vi "Clean-up List of Observables.vi"(1 "Obsv to check":string[](array[string]) caption="Quality of Run Check") -> (0 "Array":T1(array[cluster]))   [LabVIEW 2020, in "TALOS.lvlib" / "Scheduler.lvlib"]
uses:
  Scheduler.lvlib
  6c034efd-64e3-466f-95ca-04aa63bb7247.vi
  <vilib>/Comparison/Equal/Equal Functor/Equal Functor.lvclass
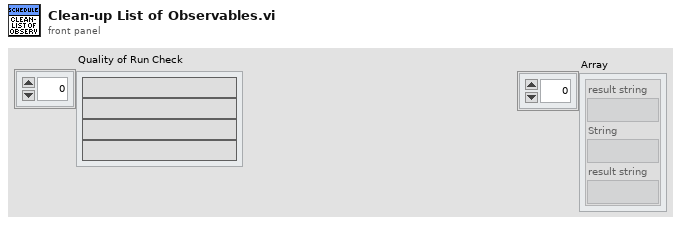
[diagram p1: front panel]
types:
  T1 = cluster{"result string":string, "String":string, "result string":string}[]
  T2 = cluster{"result string":string, "String":string, "result string":string}
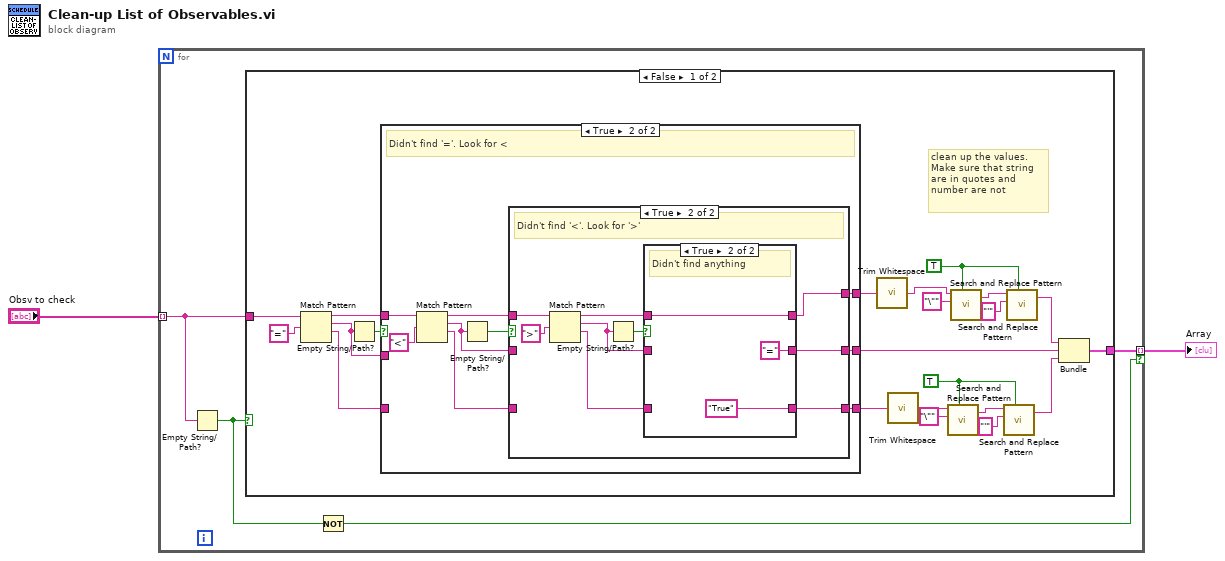
[diagram p0: block diagram]
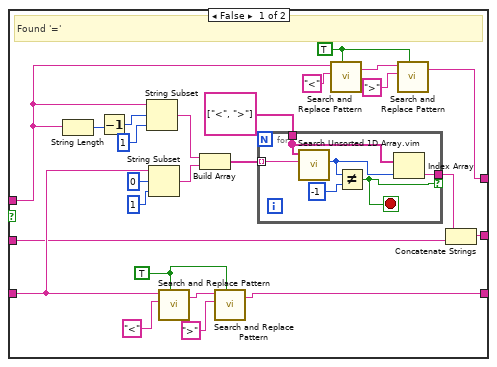
[diagram p2: hidden frame]
diagram:
  n1 = for {
    tunnel: "Obsv to check" -> [w5] mode=indexing
    tunnel: [w6] -> w2 mode=indexing if=w4
    n2 = Empty String/Path?(string/path=w5) -> (empty?=w3:bool)
    n3 = case shown="False" w3 {
      tunnel: [w11 _] -> w6
      tunnel: w5 -> [w10 _]
      frame False {
        w20 = TRUE ("replace all? (F)")
        w21 = TRUE ("replace all? (F)")
        # "clean up the values. Make sure that string are in quotes and number are not"
        n4 = Match Pattern(string=w10, regular expression="=") -> (before substring=w26:string, match substring=w15:string, after substring=w25:string)  [unwired: 1 in, 1 out]
        n5 = Empty String/Path?(string/path=w15) -> (empty?=w27:bool)
        n6 = case shown="True" w27 {
          tunnel: w26 -> [w30 w67]
          tunnel: w25 -> [w46 _]
          tunnel: [w29 w61] -> w9
          tunnel: [w48 w60] -> w16
          tunnel: w15 -> [w35 _]
          tunnel: [w37 w62] -> w13
          frame False {
            w34 = TRUE ("replace all? (F)")
            w49 = TRUE ("replace all? (F)")
            # "Found '='"
            n7 = String Length(string=w30) -> (length=w43:i32)
            n8 = Decrement(x=w43) -> (x-1=w42:i32)
            n9 = String Subset(string=w30, offset (0)=w42, length (rest)=1 ("length (rest)")) -> (substring=w41:string)
            n10 = String Subset(string=w46, offset (0)=0, length (rest)=1 ("length (rest)")) -> (substring=w40:string)
            n11 = call <vilib>:"Search and Replace Pattern.vi"("string"=w46, "regular expression (\"\")"="<" ("regular expression (\"\")"), "replace all? (F)"=w49) -> ("result string"=w52:string)  [unwired: 2 in, 1 out]
            n12 = Build Array(w41, w40) -> (w39:string[])
            n13 = call <vilib>:"Search and Replace Pattern.vi"("string"=w52, "regular expression (\"\")"=">" ("regular expression (\"\")"), "replace all? (F)"=w49) -> ("result string"=w48:string)  [unwired: 2 in, 1 out]
            n14 = for {
              tunnel: string[] ["<", ">"] -> [w56]
              tunnel: w39 -> [w58] mode=indexing
              tunnel: [w54] -> w36 if=w53
              stop <- w53 stop-if-true
              n15 = call "Search Unsorted 1D Array.vim"("element"=w58, "unsorted 1D array"=w56) -> ("index of element"=w55:i32)  [unwired: 9 in]
              n16 = Not Equal?(x=w55, y=-1) -> (x != y?=w53:bool)
              n17 = Index Array(array=w56, index=w55) -> (element=w54:string)
            }
            n18 = call <vilib>:"Search and Replace Pattern.vi"("string"=w30, "regular expression (\"\")"="<" ("regular expression (\"\")"), "replace all? (F)"=w34) -> ("result string"=w31:string)  [unwired: 2 in, 1 out]
            n19 = call <vilib>:"Search and Replace Pattern.vi"("string"=w31, "regular expression (\"\")"=">" ("regular expression (\"\")"), "replace all? (F)"=w34) -> ("result string"=w29:string)  [unwired: 2 in, 1 out]
            n20 = Concatenate Strings(w36, w35) -> (w37:string)
          }
          frame True {
            # "Didn't find '='. Look for <"
            n21 = Match Pattern(string=w67, regular expression="<") -> (before substring=w65:string, match substring=w59:string, after substring=w63:string)  [unwired: 1 in, 1 out]
            n22 = Empty String/Path?(string/path=w59) -> (empty?=w64:bool)
            n23 = case shown="True" w64 {
              tunnel: w65 -> [w69 w79]
              tunnel: w63 -> [w68 _]
              tunnel: [w70 w76] -> w62
              tunnel: [w69 w74] -> w61
              tunnel: [w68 w72] -> w60
              tunnel: w59 -> [w70 _]
              frame False {
              }
              frame True {
                # "Didn't find '<'. Look for '>'"
                n24 = Match Pattern(string=w79, regular expression=">") -> (before substring=w77:string, match substring=w73:string, after substring=w71:string)  [unwired: 1 in, 1 out]
                n25 = Empty String/Path?(string/path=w73) -> (empty?=w78:bool)
                n26 = case shown="True" w78 {
                  tunnel: w77 -> [w81 w85]
                  tunnel: [w81 w85] -> w74
                  tunnel: w73 -> [w82 _]
                  tunnel: [w82 "=" ("String")] -> w76
                  tunnel: [w80 "True"] -> w72
                  tunnel: w71 -> [w80 _]
                  frame False {
                  }
                  frame True {
                    # "Didn't find anything"
                  }
                }
              }
            }
          }
        }
        n27 = call <vilib>:"Trim Whitespace.vi"("string"=w9) -> ("trimmed string"=w8:string)  [unwired: 1 in]
        n28 = call <vilib>:"Trim Whitespace.vi"("string"=w16) -> ("trimmed string"=w7:string)  [unwired: 1 in]
        n29 = call <vilib>:"Search and Replace Pattern.vi"("string"=w7, "regular expression (\"\")"="\"" ("regular expression (\"\")"), "replace all? (F)"=w20) -> ("result string"=w17:string)  [unwired: 2 in, 1 out]
        n30 = call <vilib>:"Search and Replace Pattern.vi"("string"=w8, "regular expression (\"\")"="\"" ("regular expression (\"\")"), "replace all? (F)"=w21) -> ("result string"=w24:string)  [unwired: 2 in, 1 out]
        n31 = call <vilib>:"Search and Replace Pattern.vi"("string"=w17, "regular expression (\"\")"="'" ("regular expression (\"\")"), "replace all? (F)"=w20) -> ("result string"=w12:string)  [unwired: 2 in, 1 out]
        n32 = call <vilib>:"Search and Replace Pattern.vi"("string"=w24, "regular expression (\"\")"="'" ("regular expression (\"\")"), "replace all? (F)"=w21) -> ("result string"=w14:string)  [unwired: 2 in, 1 out]
        n33 = Bundle("result string"=w14, "String"=w13, "result string"=w12) -> (w11:T2)  [unwired: 1 in]
      }
      frame True {
        # "empty string, skip"
      }
    }
    n34 = Not(x=w3) -> (.not. x?=w4:bool)
  }
  "Array" <- w2
